vi "N5765A_Close.vi"(8 "error in (no error)":errorcluster, 11 "VISA resource name":refnum<visa-resource-name>="PS2") -> (0 "error out":errorcluster)   [LabVIEW 2015]
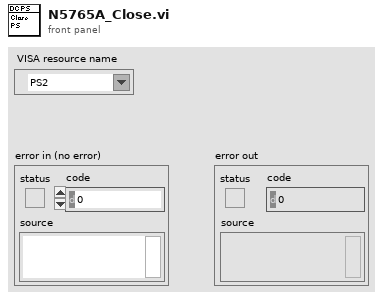
[diagram p1: front panel]
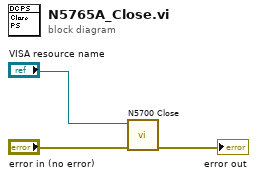
[diagram p0: block diagram]
diagram:
  n1 = call <instrlib>:"N5700 Close.vi"("error"="error in (no error)", "VISA name"="VISA resource name") -> ("error out"=→"error out":errorcluster)  [unwired: 6 in]
